vi "2D Array Zoom.vi"(7 "method":i32(ring)=2 items=["nearest", "bilinear", "bicubic", "bicubic spline"], 9 "y zoom factor":dbl=1.0, 10 "x zoom factor":dbl=1.0, 11 "Input 2D Array":dbl[][](array[numeric])) -> (1 "y dim":u32, 2 "x dim":u32, 3 "output array":dbl[][](array[numeric]))   [LabVIEW 2018]
uses:
  <vilib>/gmath/interp.llb/Interpolate 2D (1d xi,yi).vi
  <vilib>/gmath/NI_Gmath.lvlib
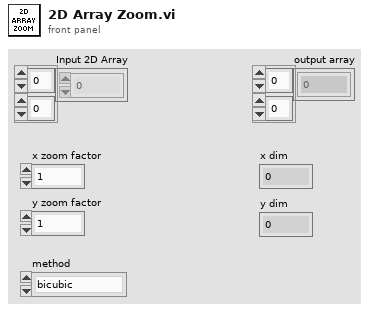
[diagram p1: front panel]
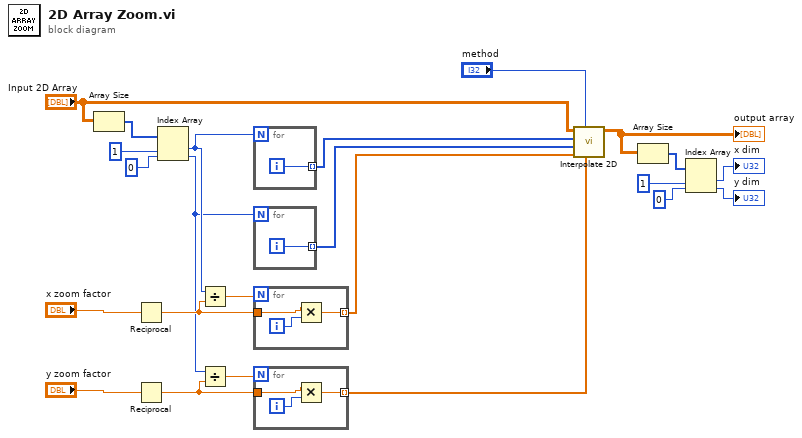
[diagram p0: block diagram]
diagram:
  n1 = Array Size(array="Input 2D Array") -> (size(s)=w15:i32[])
  n2 = Reciprocal(x="x zoom factor") -> (1/x=w6:dbl)
  n3 = Reciprocal(x="y zoom factor") -> (1/x=w5:dbl)
  n4 = Index Array(array=w15, index #1=1 ("index"), index #2=0 ("index")) -> (element #1=w4:i32, element #2=w3:i32)
  n5 = Divide(x=w4, y=w6) -> (x/y=w2:dbl)
  n6 = Divide(x=w3, y=w5) -> (x/y=w1:dbl)
  n7 = for {
    N: w4 -> [_]
    tunnel: [w24] -> w13 mode=indexing
    i -> [w24]
  }
  n8 = for {
    N: w3 -> [_]
    tunnel: [w25] -> w12 mode=indexing
    i -> [w25]
  }
  n9 = for {
    N: w2 -> [_]
    tunnel: w6 -> [w27]
    tunnel: [w26] -> w9 mode=indexing
    i -> [w28]
    n10 = Multiply(x=w27, y=w28) -> (x*y=w26:dbl)
  }
  n11 = for {
    N: w1 -> [_]
    tunnel: w5 -> [w30]
    tunnel: [w29] -> w7 mode=indexing
    i -> [w31]
    n12 = Multiply(x=w30, y=w31) -> (x*y=w29:dbl)
  }
  n13 = call-poly <vilib>:"Interpolate 2D.vi"("yi"=w7, "method"="method", "xi"=w9, "Y"=w12, "X"=w13, "Z"="Input 2D Array") -> ("zi"=w22:dbl[][])  [unwired: 2 in, 3 out]
  "output array" <- w22
  n14 = Array Size(array=w22) -> (size(s)=w21:i32[])
  n15 = Index Array(array=w21, index #1=1 ("index"), index #2=0 ("index")) -> (element #1=→"x dim":i32, element #2=→"y dim":i32)
